vi "Save Cal Data.vi"(8 "Error In":errorcluster, 10 "Scalling":T1, 11 "Config File Path":path=path "C:/Automation/Configurations/JusticeLeague.ini") -> (0 "error out":errorcluster)   [LabVIEW 2016]
uses:
  <vilib>/Utility/config.llb/Write Key (Double).vi
  <vilib>/Utility/config.llb/NI_LVConfig.lvlib
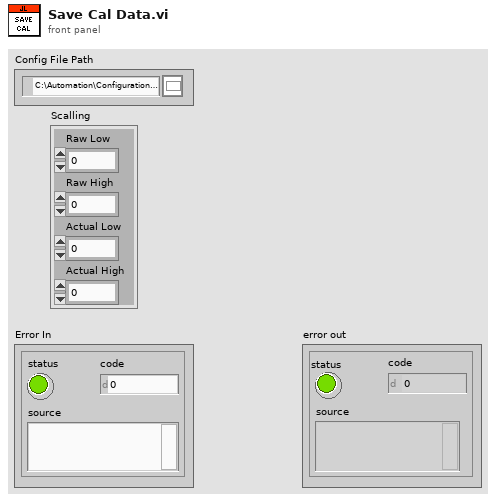
[diagram p1: front panel]
types:
  T1 = cluster{"Raw Low ":dbl, "Raw High":dbl, "Actual Low":dbl, "Actual High":dbl}
  T2 = cluster{"Calibrate?":bool, "Scalling In ":cluster{"Raw Low ":dbl, "Raw High":dbl, "Actual Low":dbl, "Actual High":dbl}}
  T3 = typedef "NI_LVConfig.lvlib/Config Data RefNum.ctl" = refnum<k1>
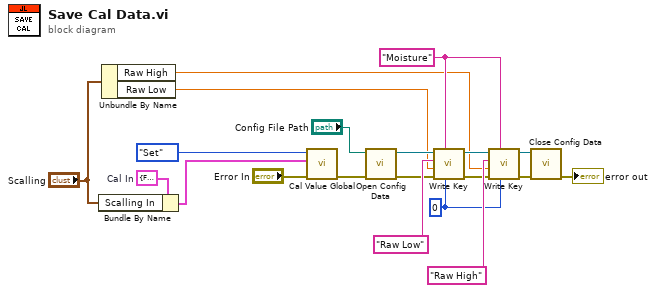
[diagram p0: block diagram]
diagram:
  w7 = T2 {"Calibrate?"=FALSE, "Scalling In "={"Raw Low "=1531.0, "Raw High"=6859.0, "Actual Low"=1.0, "Actual High"=4.9}}  # Cal In
  w9 = i16 0 ("precision (6)")
  w16 = "Moisture" ("key")
  n1 = Bundle By Name(cluster=w7, "Scalling In"="Scalling") -> (w6:T2)
  n2 = Unbundle By Name("Scalling") -> ("Raw High"=w1:dbl, "Raw Low"=w2:dbl)
  n3 = call "Cal Value Global.vi"("error in (no error)"="Error In", "Cal In"=w6, "Action"=enum16{"Set", "Get "}."Set") -> ("error out"=w3:errorcluster)  [unwired: 7 in, 1 out]
  n4 = call <vilib>:"Open Config Data.vi"("error in (no error)"=w3, "configuration file path"="Config File Path") -> ("error out"=w14:errorcluster, "refnum"=w19:T3)  [unwired: 7 in, 1 out]
  n5 = call-poly <vilib>:"Write Key.vi"("precision (6)"=w9, "section"=w16, "error in (no error)"=w14, "value"=w2, "key"="Raw Low", "refnum"=w19) -> ("error out"=w13:errorcluster, "refnum out"=w18:T3)  [unwired: 3 in, 1 out]
  n6 = call-poly <vilib>:"Write Key.vi"("precision (6)"=w9, "section"=w16, "error in (no error)"=w13, "value"=w1, "key"="Raw High", "refnum"=w18) -> ("error out"=w11:errorcluster, "refnum out"=w12:T3)  [unwired: 3 in, 1 out]
  n7 = call <vilib>:"Close Config Data.vi"("error in (no error)"=w11, "refnum"=w12) -> ("error out"=→"error out":errorcluster)  [unwired: 8 in, 1 out]
